vi "Standartteil.vi"(7 "error in (no error)":errorcluster caption="Fehler (Eingang, kein Fehler)", 10 "Device ID":T1(ring)) -> (0 "error out":errorcluster caption="Fehler (Ausgang)")   [LabVIEW 2010]
uses:
  globale Variable 1.vi
panel:
  out "Numerisches Element":i32
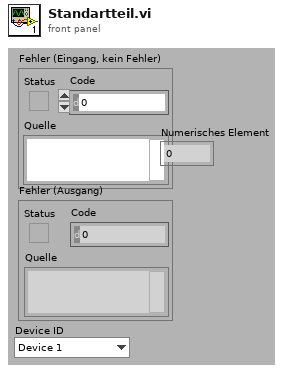
[diagram p1: front panel]
types:
  T1 = enum16{"Device 1", "Device 2", "Device 3", "Device 4", "Device 5", "Device 6", "Device 7", "Device 8"}
  T2 = enum8{"Robo Interface", "Extension 1", "Extension 2", "Extension 3"}
  T3 = enum8{"Output 1 (O1)", "Output 2 (O2)", "Output 3 (O3)", "Output 4 (O4)", "Output 5 (O5)", "Output 6 (O6)", "Output 7 (O7)", "Output 8 (O8)"}
  T4 = enum8{"Power 1", "Power 2", "Power 3", "Power 4", "Power 5", "Power 6", "Power 7", "Power 8"}
  T5 = enum8{"Goes High", "Goes Low", "Goes High or Low"}
  T6 = enum8{"Input 1 (I1)", "Input 2 (I2)", "Input 3 (I3)", "Input 4 (I4)", "Input 5 (I5)", "Input 6 (I6)", "Input 7 (I7)", "Input 8 (I8)"}
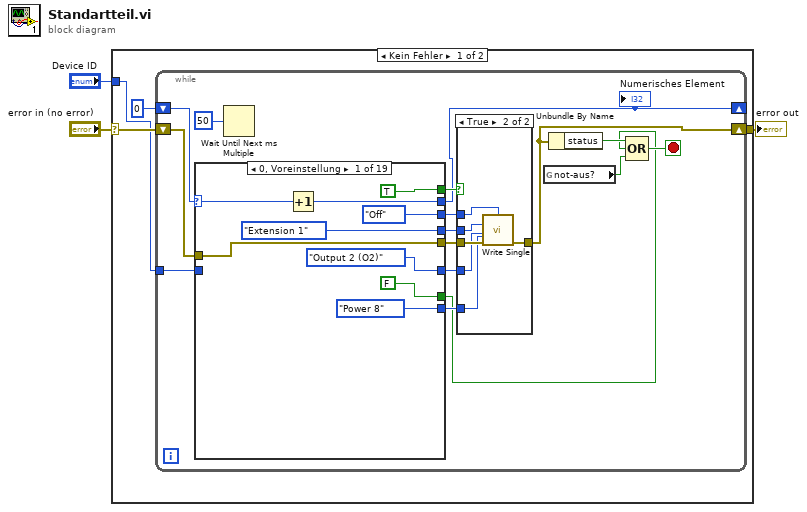
[diagram p0: block diagram]
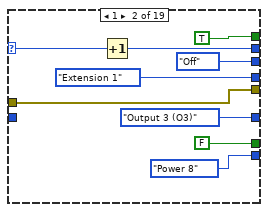
[diagram p3: hidden frame]
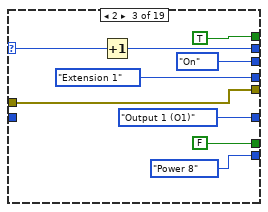
[diagram p4: hidden frame]
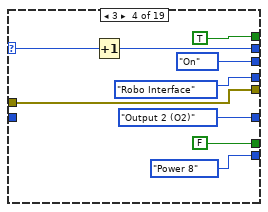
[diagram p5: hidden frame]
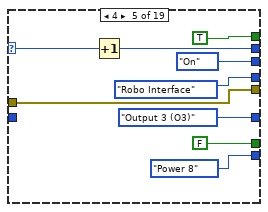
[diagram p6: hidden frame]
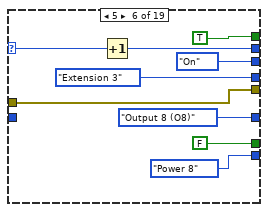
[diagram p7: hidden frame]
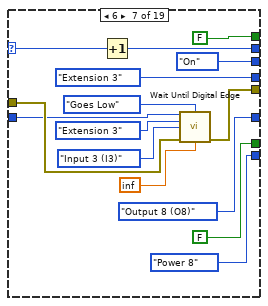
[diagram p8: hidden frame]
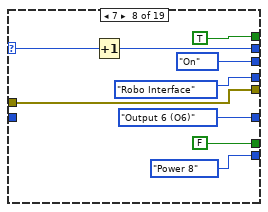
[diagram p9: hidden frame]
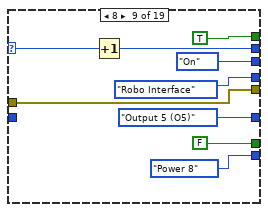
[diagram p10: hidden frame]
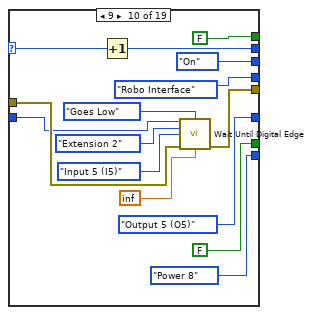
[diagram p11: hidden frame]
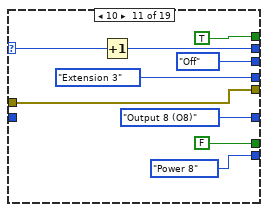
[diagram p12: hidden frame]
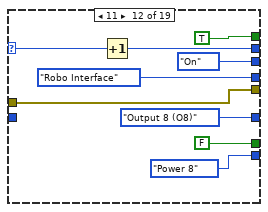
[diagram p13: hidden frame]
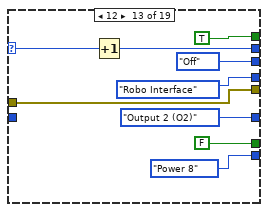
[diagram p14: hidden frame]
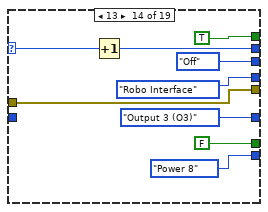
[diagram p15: hidden frame]
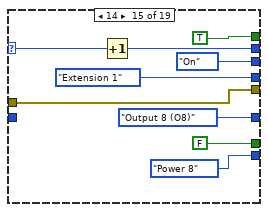
[diagram p16: hidden frame]
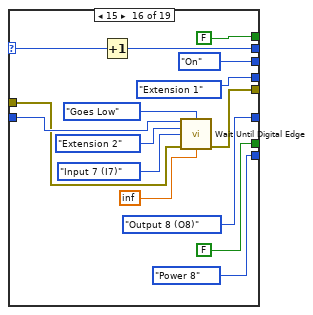
[diagram p17: hidden frame]
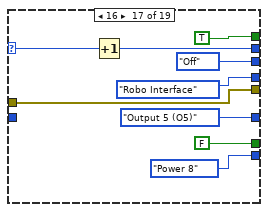
[diagram p18: hidden frame]
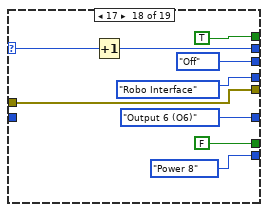
[diagram p19: hidden frame]
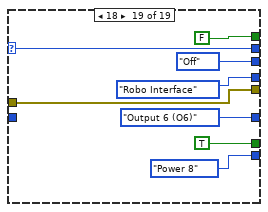
[diagram p20: hidden frame]
diagram:
  n1 = case shown="Kein Fehler" "error in (no error)" {
    selector: "error in (no error)" -> [w7 w219]
    tunnel: "Device ID" -> [w6 _]
    tunnel: [w5 w219] -> w1
    frame No Error {
      n2 = while {
        shift-right: [w14] -> w5
        shift-left: w7 -> [w13]
        tunnel: w6 -> [w12]
        shift-right: [w8] -> _
        shift-left: 0 -> [w11]
        stop <- w21 stop-if-true
        n3 = case shown="0, Voreinstellung" w11 {
          selector: w11 -> [w34 w43 w52 w61 w70 w79 w94 w103 w112 w127 w136 w145 w154 w163 w172 w187 w196 w205 w212]
          tunnel: [T4."Power 8" ("Output_PWM") T4."Power 8" ("Output_PWM") T4."Power 8" ("Output_PWM") T4."Power 8" ("Output_PWM") T4."Power 8" ("Output_PWM") T4."Power 8" ("Output_PWM") T4."Power 8" ("Output_PWM") T4."Power 8" ("Output_PWM") T4."Power 8" ("Output_PWM") T4."Power 8" ("Output_PWM") T4."Power 8" ("Output_PWM") T4."Power 8" ("Output_PWM") T4."Power 8" ("Output_PWM") T4."Power 8" ("Output_PWM") T4."Power 8" ("Output_PWM") T4."Power 8" ("Output_PWM") T4."Power 8" ("Output_PWM") T4."Power 8" ("Output_PWM") T4."Power 8" ("Output_PWM")] -> w19
          tunnel: [T3."Output 2 (O2)" ("Single_Output") T3."Output 3 (O3)" ("Single_Output") T3."Output 1 (O1)" ("Single_Output") T3."Output 2 (O2)" ("Single_Output") T3."Output 3 (O3)" ("Single_Output") T3."Output 8 (O8)" ("Single_Output") T3."Output 8 (O8)" ("Single_Output") T3."Output 6 (O6)" ("Single_Output") T3."Output 5 (O5)" ("Single_Output") T3."Output 5 (O5)" ("Single_Output") T3."Output 8 (O8)" ("Single_Output") T3."Output 8 (O8)" ("Single_Output") T3."Output 2 (O2)" ("Single_Output") T3."Output 3 (O3)" ("Single_Output") T3."Output 8 (O8)" ("Single_Output") T3."Output 8 (O8)" ("Single_Output") T3."Output 5 (O5)" ("Single_Output") T3."Output 6 (O6)" ("Single_Output") T3."Output 6 (O6)" ("Single_Output")] -> w16
          tunnel: [enum8{"Off", "On"}."Off" ("Output_Action") enum8{"Off", "On"}."Off" ("Output_Action") enum8{"Off", "On"}."On" ("Output_Action") enum8{"Off", "On"}."On" ("Output_Action") enum8{"Off", "On"}."On" ("Output_Action") enum8{"Off", "On"}."On" ("Output_Action") enum8{"Off", "On"}."On" ("Output_Action") enum8{"Off", "On"}."On" ("Output_Action") enum8{"Off", "On"}."On" ("Output_Action") enum8{"Off", "On"}."On" ("Output_Action") enum8{"Off", "On"}."Off" ("Output_Action") enum8{"Off", "On"}."On" ("Output_Action") enum8{"Off", "On"}."Off" ("Output_Action") enum8{"Off", "On"}."Off" ("Output_Action") enum8{"Off", "On"}."On" ("Output_Action") enum8{"Off", "On"}."On" ("Output_Action") enum8{"Off", "On"}."Off" ("Output_Action") enum8{"Off", "On"}."Off" ("Output_Action") enum8{"Off", "On"}."Off" ("Output_Action")] -> w18
          tunnel: [T2."Extension 1" ("Module") T2."Extension 1" ("Module") T2."Extension 1" ("Module") T2."Robo Interface" ("Module") T2."Robo Interface" ("Module") T2."Extension 3" ("Module") T2."Extension 3" ("Module") T2."Robo Interface" ("Module") T2."Robo Interface" ("Module") T2."Robo Interface" ("Module") T2."Extension 3" ("Module") T2."Robo Interface" ("Module") T2."Robo Interface" ("Module") T2."Robo Interface" ("Module") T2."Extension 1" ("Module") T2."Extension 1" ("Module") T2."Robo Interface" ("Module") T2."Robo Interface" ("Module") T2."Robo Interface" ("Module")] -> w17
          tunnel: [TRUE TRUE TRUE TRUE TRUE TRUE FALSE TRUE TRUE FALSE TRUE TRUE TRUE TRUE TRUE FALSE TRUE TRUE FALSE] -> w15
          tunnel: [FALSE FALSE FALSE FALSE FALSE FALSE FALSE FALSE FALSE FALSE FALSE FALSE FALSE FALSE FALSE FALSE FALSE FALSE TRUE] -> w9
          tunnel: [w33 w42 w51 w60 w69 w78 w93 w102 w111 w126 w135 w144 w153 w162 w171 w186 w195 w204 w212] -> w8
          tunnel: [w31 w40 w49 w58 w67 w76 w87 w100 w109 w124 w133 w142 w151 w160 w169 w184 w193 w202 w211] -> w20
          tunnel: w12 -> [_ _ _ _ _ _ w85 _ _ w118 _ _ _ _ _ w180 _ _ _]
          tunnel: w13 -> [w31 w40 w49 w58 w67 w76 w86 w100 w109 w119 w133 w142 w151 w160 w169 w178 w193 w202 w211]
          frame 0, Default {
            n4 = Increment(x=w34) -> (x+1=w33:i32)
          }
          frame 1 {
            n5 = Increment(x=w43) -> (x+1=w42:i32)
          }
          frame 2 {
            n6 = Increment(x=w52) -> (x+1=w51:i32)
          }
          frame 3 {
            n7 = Increment(x=w61) -> (x+1=w60:i32)
          }
          frame 4 {
            n8 = Increment(x=w70) -> (x+1=w69:i32)
          }
          frame 5 {
            n9 = Increment(x=w79) -> (x+1=w78:i32)
          }
          frame 6 {
            n10 = Increment(x=w94) -> (x+1=w93:i32)
            n11 = call "Wait Until Digital Edge.vi"("Device ID"=w85, "Wait Until"=T5."Goes Low", "Module"=T2."Extension 3", "Digital_Input"=T6."Input 3 (I3)", "error in"=w86, "Time Out (10)"=inf) -> ("error out"=w87:errorcluster)  [unwired: 9 out]
          }
          frame 7 {
            n12 = Increment(x=w103) -> (x+1=w102:i32)
          }
          frame 8 {
            n13 = Increment(x=w112) -> (x+1=w111:i32)
          }
          frame 9 {
            n14 = Increment(x=w127) -> (x+1=w126:i32)
            n15 = call "Wait Until Digital Edge.vi"("Device ID"=w118, "Wait Until"=T5."Goes Low", "Module"=T2."Extension 2", "Digital_Input"=T6."Input 5 (I5)", "error in"=w119, "Time Out (10)"=inf) -> ("error out"=w124:errorcluster)  [unwired: 9 out]
          }
          frame 10 {
            n16 = Increment(x=w136) -> (x+1=w135:i32)
          }
          frame 11 {
            n17 = Increment(x=w145) -> (x+1=w144:i32)
          }
          frame 12 {
            n18 = Increment(x=w154) -> (x+1=w153:i32)
          }
          frame 13 {
            n19 = Increment(x=w163) -> (x+1=w162:i32)
          }
          frame 14 {
            n20 = Increment(x=w172) -> (x+1=w171:i32)
          }
          frame 15 {
            n21 = Increment(x=w187) -> (x+1=w186:i32)
            n22 = call "Wait Until Digital Edge.vi"("Device ID"=w180, "Wait Until"=T5."Goes Low", "Module"=T2."Extension 2", "Digital_Input"=T6."Input 7 (I7)", "error in"=w178, "Time Out (10)"=inf) -> ("error out"=w184:errorcluster)  [unwired: 9 out]
          }
          frame 16 {
            n23 = Increment(x=w196) -> (x+1=w195:i32)
          }
          frame 17 {
            n24 = Increment(x=w205) -> (x+1=w204:i32)
          }
          frame 18 {
          }
        }
        "Numerisches Element" <- w8
        n25 = Wait Until Next ms Multiple(millisecond multiple=50) -> ()  [unwired: 1 out]
        n26 = case shown="TRUE" w15 {
          tunnel: [w24 w30] -> w14
          tunnel: w20 -> [w24 w29]
          tunnel: w16 -> [_ w28]
          tunnel: w17 -> [_ w27]
          tunnel: w18 -> [_ w26]
          tunnel: w19 -> [_ w25]
          frame False {
          }
          frame True {
            n27 = call "Write Single.vi"("Output_Action"=w26, "Module"=w27, "Single_Output"=w28, "Output_PWM"=w25, "error in"=w29) -> ("error out"=w30:errorcluster)  [unwired: 1 in, 9 out]
          }
        }
        n28 = global read "globale Variable 1.vi" "not-aus?"() -> (w10:bool)
        n29 = Unbundle By Name(w14) -> ("status"=w22:bool)
        n30 = Compound Arithmetic op=OR(w22, w9, w10) -> (w21:bool)
      }
    }
    frame Error {
    }
  }
  "error out" <- w1
